vi "PicohrdlSetDigitalIOChannel.vi"(7 "digitalOutPinState":i16, 8 "error in (no error)":errorcluster, 11 "Handle in":i16) -> (0 "error out":errorcluster, 3 "Handle out":i16, 6 "digitalOutPinState(out)":i16)   [LabVIEW 2010]
uses:
  PicoHRDL.dll
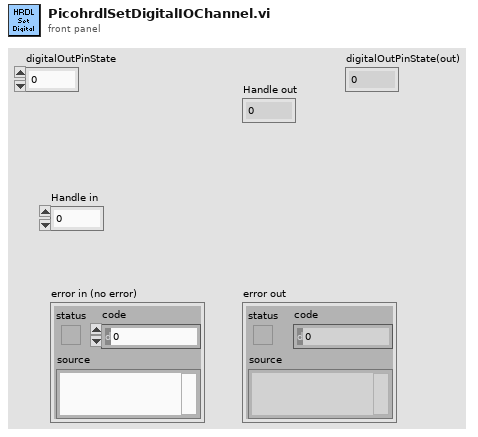
[diagram p1: front panel]
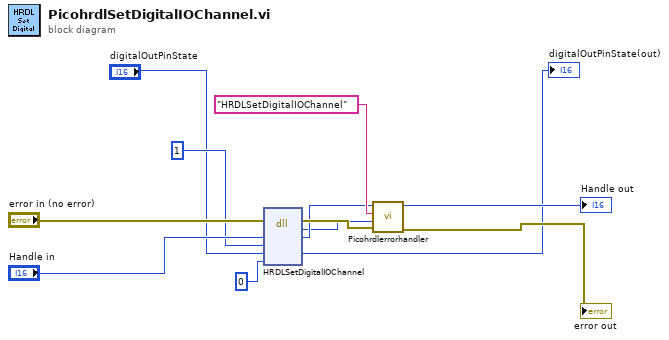
[diagram p0: block diagram]
diagram:
  n1 = dll-call lib="PicoHRDL.dll" fn="HRDLSetDigitalIOChannel"(error in="error in (no error)", "handle"="Handle in", "directionOut"=i16 1, "digitalOutPinState"="digitalOutPinState", "enabledDigitalIn"=i16 0) -> (error out=w7:errorcluster, "return type"=w5:i16, "handle"=w6:i16, "digitalOutPinState"=→"digitalOutPinState(out)":i16)  [unwired: 4 in, 1 out]
  n2 = call "Picohrdlerrorhandler.vi"("Handle in"=w6, "API function"="HRDLSetDigitalIOChannel", "Return"=w5, "error in (no error)"=w7) -> ("Handle out"=→"Handle out":i16, "error out"=→"error out":errorcluster)  [unwired: 5 in]
